vi "Write Current State Msg.vi"(8 "error in (no error)":errorcluster, 10 "Elevator.lvlib:Current State Msg.lvclass":refnum<class "Current State Msg.lvclass">, 11 "Request Current State Msg in":refnum<class "Request Current State Msg.lvclass">) -> (0 "error out":errorcluster, 3 "Request Current State Msg out":refnum<class "Request Current State Msg.lvclass">)   [LabVIEW 2014, in "Elevator.lvlib" / "Request Current State Msg.lvclass"]
uses:
  Request Current State Msg.lvclass
  Current State Msg/Current State Msg.lvclass
  Request Current State Msg.lvclass/Request Current State Msg.ctl
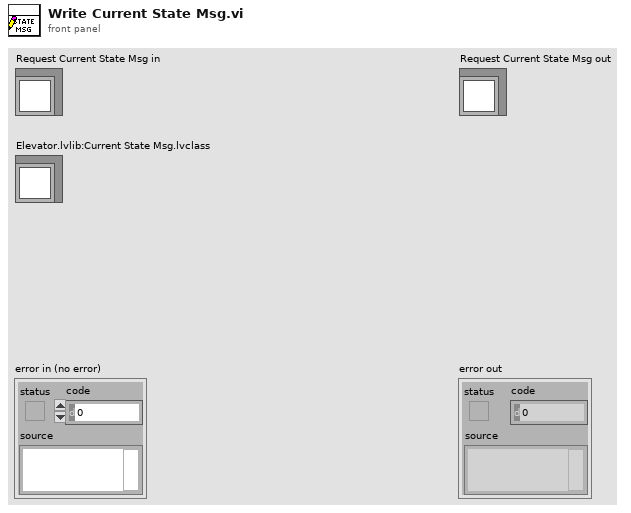
[diagram p1: front panel]
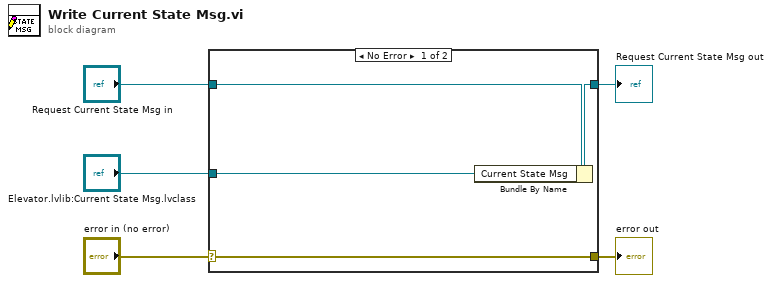
[diagram p0: block diagram]
diagram:
  n1 = case shown="No Error" "error in (no error)" {
    selector: "error in (no error)" -> [w9 w10]
    tunnel: [w9 w10] -> w4
    tunnel: [w7 w11] -> w2
    tunnel: "Request Current State Msg in" -> [w8 w11]
    tunnel: "Elevator.lvlib:Current State Msg.lvclass" -> [w6 _]
    frame No Error {
      n2 = Bundle By Name(cluster=w8, "Current State Msg"=w6) -> (w7:refnum<class "Request Current State Msg.lvclass">)
    }
    frame Error {
    }
  }
  "error out" <- w4
  "Request Current State Msg out" <- w2
